vi "Create A New Group.vi"(4 "error in (no error)":errorcluster, 5 "Axis Number":i32[](array[numeric])=[1, 2] min=1 max=3 format="%#.0f", 6 "Group Number (1)":i32=1 min=1, 7 "VISA resource name":refnum<visa-resource-name>="COM5") -> (0 "error out":errorcluster, 3 "VISA resource name out":refnum<visa-resource-name>="COM5")   [LabVIEW 2019, in "Newport ESP301.lvlib"]
doc: "This command (HN) is used to create a new group. A few rules are in place to facilitate easy management of groups.\n• A group has to be created with at least two axes assigned to it before any command related to groups can be issued. The controller returns error 15, GROUP NUMBER NOT ASSIGNED, if, for instance, one tries to set velocity for group #1, before creating group #1.\n• A group has to be deleted (refer HX command) before axes assigned to the group can be changed. The controller returns error 16, GROUP NUMBER ALREADY ASSIGNED, if one attempts to change axes assigned to a group already created. Please see the following table for correct method to change axes assigned to a group:\nCorrect Method Incorrect Method\n1HN1,2 1HN2,3\n1HN1,2 1HN2,3\n1HX\n• An axis cannot be a member of (or assigned to) different groups at the same time. The controller returns error 18, GROUP AXIS ALREADY ASSIGNED, if one attempts to assign an axis under such circumstances. Refer HX command to delete a group.\n• An axis cannot be assigned more than once in a group. The controller returns error 19, GROUP AXIS DUPLICATED, if one attempts to assign an axis more than once to a group.\n• The order in which axes are assigned to a group is very important. This is because it specifies the frame of reference in which coordinated motion of axes takes place. For instance, the command 1HN1,2 assigns axis numbers 1 and 2 to group number 1, where axis #1 is equivalent to X-axis and axis #2 is equivalent to Y-axis in a traditional cartesian coordinate system. Reversing the ordering of axes (viz. 1HN2,1) reverses the axis assignment.\n• If a group has more than two axes assigned to it, and the group was commanded to make an arc (refer to HC command), the first two axes in the group are used to make the desired move."
uses:
  Newport ESP301.lvlib
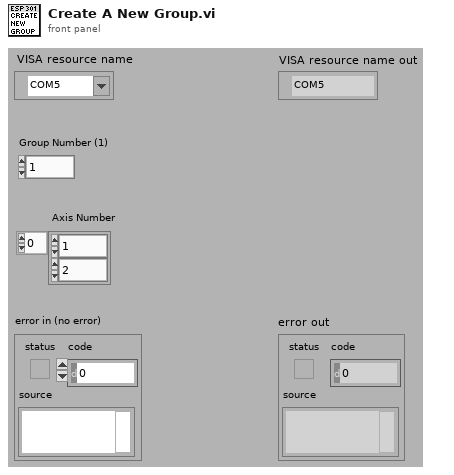
[diagram p1: front panel]
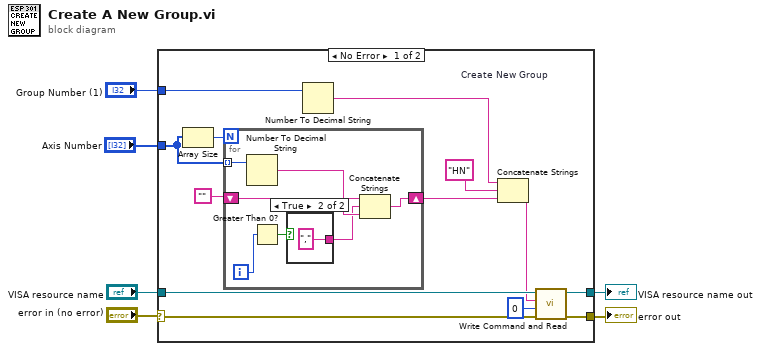
[diagram p0: block diagram]
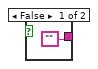
[diagram p2: hidden frame]
diagram:
  n1 = case shown="No Error" "error in (no error)" {
    selector: "error in (no error)" -> [w16 w30]
    tunnel: [w18 w30] -> w6
    tunnel: "VISA resource name" -> [w19 w29]
    tunnel: [w17 w29] -> w5
    tunnel: "Group Number (1)" -> [w14 _]
    tunnel: "Axis Number" -> [w10 _]
    frame No Error {
      w12 = "HN"  # Create New Group
      n2 = Array Size(array=w10) -> (size(s)=w9:i32)
      n3 = for {
        N: w9 -> [_]
        tunnel: w10 -> [w26] mode=indexing
        shift-right: [w24] -> w7
        shift-left: "" -> [w23]
        i -> [w21]
        n4 = Number To Decimal String(number=w26) -> (decimal integer string=w25:string)  [unwired: 1 out]
        n5 = Greater Than 0?(x=w21) -> (x > 0?=w20:bool)
        n6 = case shown="True" w20 {
          tunnel: ["" "," ("séparateur (Tabulation)")] -> w22
          frame False {
          }
          frame True {
          }
        }
        n7 = Concatenate Strings(w23, w22, w25) -> (w24:string)
      }
      n8 = Number To Decimal String(number=w14) -> (decimal integer string=w11:string)  [unwired: 1 out]
      n9 = Concatenate Strings(w11, w12, w7) -> (w15:string)
      n10 = call "Write Command and Read.vi"("error in (no error)"=w16, "Bytes to read (100)"=u32 0, "Command"=w15, "VISA resource name"=w19) -> ("error out"=w18:errorcluster, "VISA resource name out"=w17:refnum<visa-resource-name>)  [unwired: 1 in, 3 out]
    }
    frame Error {
    }
  }
  "error out" <- w6
  "VISA resource name out" <- w5
